vi "Save Document.vi"(8 "error in (no error)":errorcluster, 11 "Document API in":refnum<class "Document API.lvclass">) -> (0 "error out":errorcluster, 3 "Document API out":refnum<class "Document API.lvclass">)   [LabVIEW 2017, in "Document API.lvlib" / "Document API.lvclass"]
doc: "Saves the <b>Document in</b> to the <b>Document Path</b> location given in the create or open method. Use get document path to retrieve the saved file location.\n\nNotes:\n - If <b>Document Path</b> is empty or is <Not A Path> or is a directory, the VI saves the document at a generated file path into the temporary directory."
uses:
  Document API.lvclass
  Document API.lvclass/Document API.ctl
  NPOI_Document/npoiDocument/npoiDocument.lvclass
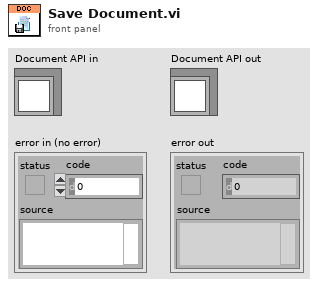
[diagram p1: front panel]
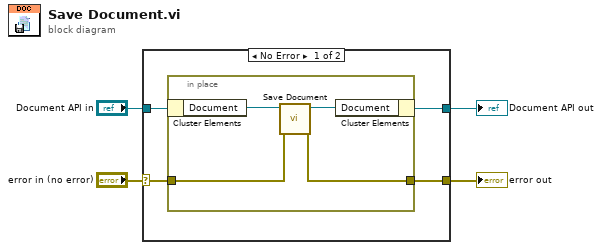
[diagram p0: block diagram]
diagram:
  n1 = case shown="No Error" "error in (no error)" {
    selector: "error in (no error)" -> [w6 w14]
    tunnel: [w5 w14] -> w3
    tunnel: [w8 w13] -> w1
    tunnel: "Document API in" -> [w7 w13]
    frame No Error {
      n2 = in-place {
        in-place-border: w6 -> [w10]
        in-place-border: [w9] -> w5
        n3 = in-place-cluster #1(w7) -> ("Document"=w12:refnum<class "npoiDocument.lvclass">)
        n4 = call "Save Document.vi"("error in (no error)"=w10, "Document in"=w12) -> ("error out"=w9:errorcluster, "Document out"=w11:refnum<class "npoiDocument.lvclass">)  [unwired: 8 in]
        n5 = in-place-cluster #1("Document"=w11) -> (w8:refnum<class "Document API.lvclass">)
      }
    }
    frame Error {
    }
  }
  "error out" <- w3
  "Document API out" <- w1
